vi "Creat.vi"(8 "error in (no error)":errorcluster, 10 "mode path":path) -> (0 "error out":errorcluster, 3 "FaceRecognition out":refnum<class "FaceRecognition.lvclass">)   [LabVIEW 2020, in "FaceRecognitionDotNet.lvlib" / "FaceRecognition.lvclass"]
uses:
  FaceRecognition.lvclass
  dll/FaceRecognitionDotNet.dll
  FaceRecognition.lvclass/FaceRecognition.ctl
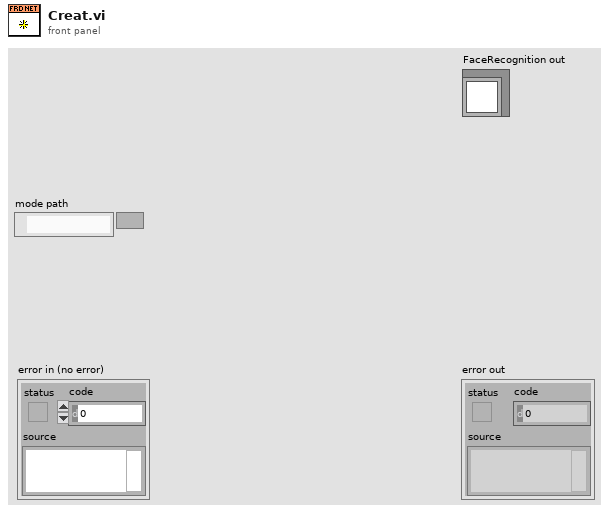
[diagram p1: front panel]
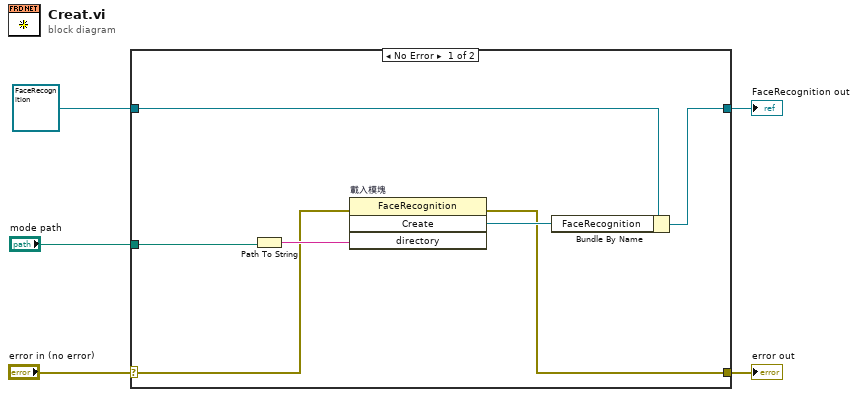
[diagram p0: block diagram]
diagram:
  n1 = case shown="No Error" "error in (no error)" {
    selector: "error in (no error)" -> [w10 w14]
    tunnel: [w7 w14] -> w4
    tunnel: [w9 w13] -> w2
    tunnel: refnum<class "FaceRecognition.lvclass"> refnum ("FaceRecognition in") -> [w6 w13]
    tunnel: "mode path" -> [w12 _]
    frame No Error {
      n2 = Path To String(path=w12) -> (string=w11:string)
      n3 = invoke on="載入模塊" class="FaceRecognition" method="Create"(error in=w10, "directory"=w11) -> (error out=w7:errorcluster, "Create"=w8:refnum<k24>)  [unwired: 2 in, 2 out]
      n4 = Bundle By Name(cluster=w6, "FaceRecognition"=w8) -> (w9:refnum<class "FaceRecognition.lvclass">)
    }
    frame Error {
    }
  }
  "error out" <- w4
  "FaceRecognition out" <- w2
